vi "epx_Vector.Width Write.vi"(4 "error in (no error)":errorcluster, 5 "Value":u8, 6 "Container State":T3, 7 "Display State In":T1={"BGColor"=16448250, "FGColor"=0, "GridColor"=9868950, "Number of Polar Grids"=12, "Number of Circle Grids"=4, "Vector.Active"=0, "Vectors.Properties"=[], "Height"=300, "Width"=300} {"Number of Circle Grids" min=1 max=100 step=1; "Number of Polar Grids" min=1 max=100 step=1}) -> (0 "error out":errorcluster, 3 "Display State Out":T1={"BGColor"=16448250, "FGColor"=0, "GridColor"=9868950, "Number of Polar Grids"=12, "Number of Circle Grids"=4, "Vector.Active"=0, "Vectors.Properties"=[], "Height"=300, "Width"=300} {"Number of Circle Grids" min=1 max=100 step=1; "Number of Polar Grids" min=1 max=100 step=1})   [LabVIEW 2011, in "NI_EP_Basic.lvlib" / "EPX Vector Diagram.xctl"]
uses:
  <vilib>/addons/Electrical Power/Basic/Controls/Vector Diagram/EPX Vector Diagram.xctl
  <vilib>/_xctls/Container State.ctl
  <vilib>/addons/Electrical Power/Basic/Controls/Vector Diagram/Abilities/epx_Vector Diagram State.ctl
  <vilib>/addons/Electrical Power/Basic/Controls/Vector Diagram/SubVIs/epx_Vector Type.ctl
  <vilib>/_xctls/XControlSupport.lvlib
  <vilib>/addons/Electrical Power/Basic/NI_EP_Basic.lvlib
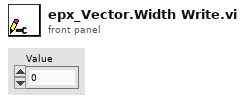
[diagram p1: front panel]
types:
  T1 = typedef "NI_EP_Basic.lvlib/EPX Vector Diagram.xctl/epx_Vector Diagram State.ctl" = cluster{"BGColor":u32, "FGColor":u32, "GridColor":u32, "Number of Polar Grids":i32, "Number of Circle Grids":i32, "Vector.Active":i32, "Vectors.Properties":cluster{"Vector.Type":T2, "Vector.Color":u32, "Vector.Width":u8}[], "Height":u32, "Width":u32}
  T2 = typedef "NI_EP_Basic.lvlib/epx_Vector Type.ctl" = enum16{"Voltage", "Current"}
  T3 = typedef "XControlSupport.lvlib/Container State.ctl" = cluster{"Indicator?":bool, "Run Mode?":bool, " Refnum":refnum<vi>}
  T4 = cluster{"Vector.Type":T2, "Vector.Color":u32, "Vector.Width":u8}[]
  T5 = cluster{"Vector.Type":T2, "Vector.Color":u32, "Vector.Width":u8}
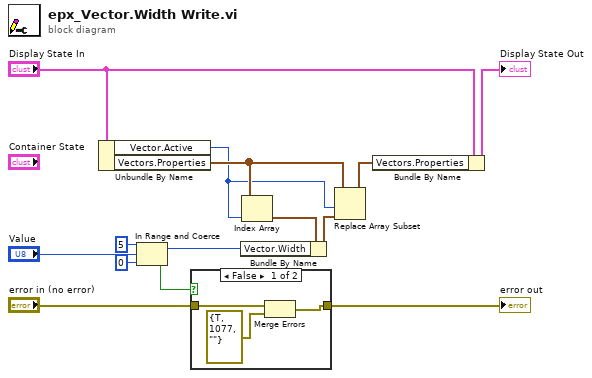
[diagram p0: block diagram]
diagram:
  n1 = Unbundle By Name("Display State In") -> ("Vector.Active"=w12:i32, "Vectors.Properties"=w13:T4)
  n2 = In Range and Coerce(upper limit=u8 5, x="Value", lower limit=u8 0) -> (coerced(x)=w2:u8, In Range?=w1:bool)
  n3 = case shown="False" w1 {
    tunnel: [w17 w18] -> w5
    tunnel: "error in (no error)" -> [w16 w18]
    frame False {
      n4 = Merge Errors(w16, errorcluster {"status"=TRUE, "code"=1077, "source"=""} ("error in")) -> (w17:errorcluster)
    }
    frame True {
    }
  }
  "error out" <- w5
  n5 = Index Array(array=w13, index=w12) -> (element=w14:T5)
  n6 = Bundle By Name(cluster=w14, "Vector.Width"=w2) -> (w10:T5)
  n7 = Replace Array Subset(array=w13, new element=w10, index=w12) -> (w11:T4)
  n8 = Bundle By Name(cluster="Display State In", "Vectors.Properties"=w11) -> (→"Display State Out":T1)
